vi "connect.vi"(0 "reference":refnum<class "StateDiagramGraph.lvclass">, 1 "egde":refnum<class "AbstractEdge.lvclass">, 2 "2dPoint1":T1 {"y" format="%.2f"; "x" format="%.2f"}, 3 "2dPoint2":T1 {"y" format="%.2f"; "x" format="%.2f"}, 5 "error in (no error)":errorcluster) -> (14 "reference out":refnum<class "StateDiagramGraph.lvclass">, 15 "connected":bool, 19 "error out":errorcluster)   [LabVIEW 2020, in "StateDiagramGraph.lvclass"]
doc: "/**\n A UML class diagram.\n*/\npublic class StateDiagramGraph extends Graph"
uses:
  <resource>/Framework/Providers/Open_GDS/UML/StateDiagramGraph_class/StateDiagramGraph.lvclass
  <resource>/Framework/Providers/Open_GDS/UML/AbstractEdge_class/AbstractEdge.lvclass
  <resource>/Framework/Providers/Open_GDS/UML/General/Point/Point Point2D.ctl
  <resource>/Framework/Providers/Open_GDS/UML/Graph_class/Graph.lvclass
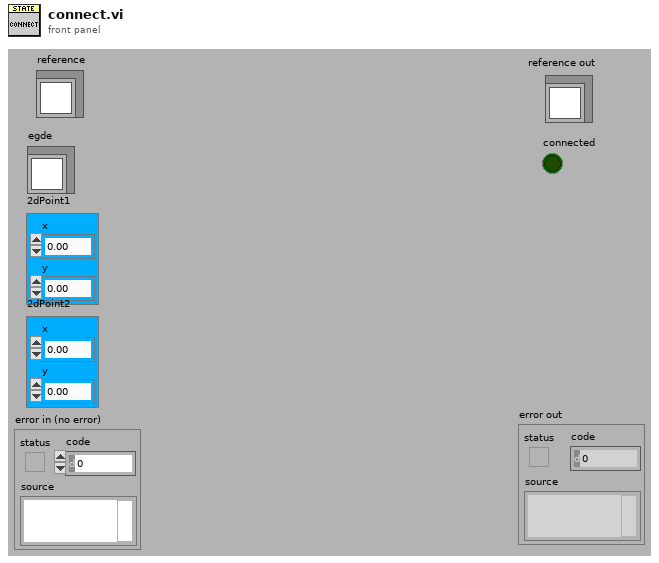
[diagram p1: front panel]
types:
  T1 = typedef "Point Point2D.ctl" = cluster{"x":dbl, "y":dbl}
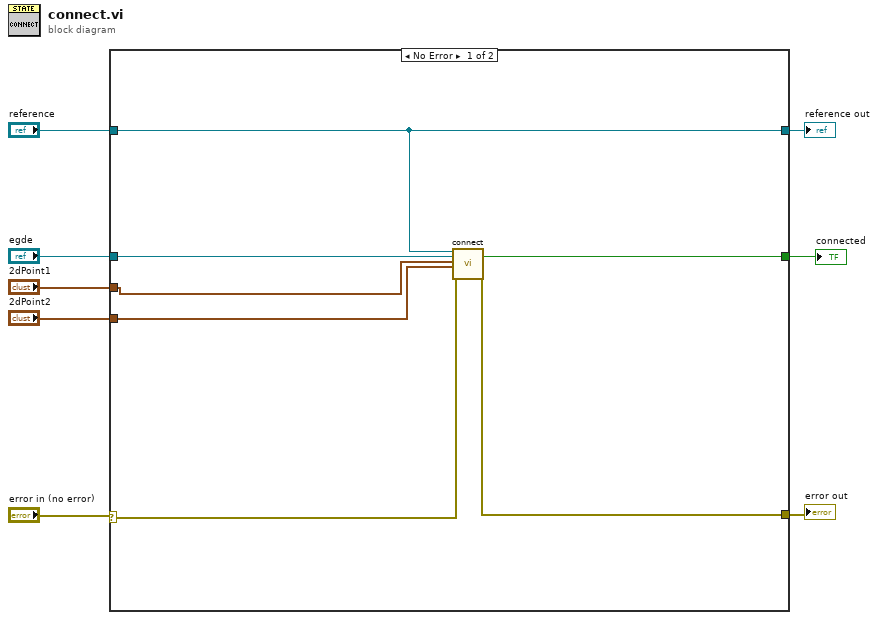
[diagram p0: block diagram]
diagram:
  n1 = case shown="No Error" "error in (no error)" {
    selector: "error in (no error)" -> [w11 w16]
    tunnel: "reference" -> [w15 w17]
    tunnel: [w10 w16] -> w7
    tunnel: [w15 w17] -> w6
    tunnel: "egde" -> [w14 _]
    tunnel: "2dPoint1" -> [w13 _]
    tunnel: "2dPoint2" -> [w12 _]
    tunnel: [w9 _] -> w1
    frame No Error {
      n2 = call-parent "connect.vi"("reference"=w15, "egde"=w14, "p1"=w13, "p2"=w12, "error in (no error)"=w11) -> ("connected"=w9:bool, "error out"=w10:errorcluster)  [unwired: 12 in, 1 out]
    }
    frame Error {
    }
  }
  "reference out" <- w6
  "error out" <- w7
  "connected" <- w1
